vi "createState.vi"(8 "error in (no error)":errorcluster, 10 "State:":T1, 11 "StateFactory in":refnum<class "StateFactory.lvclass">) -> (0 "error out":errorcluster, 2 "State.lvclass":refnum<class "State.lvclass">, 3 "StateFactory out":refnum<class "StateFactory.lvclass">)   [LabVIEW 2015, in "StateFactory.lvclass"]
uses:
  StateFactory.lvclass
  Typedefs/StateSelector.ctl
  State/State.lvclass
  States/OfflineState/OfflineState.lvclass
  States/FaultState/FaultState.lvclass
  States/StandbyState/StandbyState.lvclass
  States/DisabledState/DisabledState.lvclass
  States/EnabledState/EnabledState.lvclass
  States/WaitForUserInputState/WaitForUserInputState.lvclass
  States/PerformOpenLoopScanState/PerformOpenLoopScanState.lvclass
  States/PerformClosedLoopScanState/PerformClosedLoopScanState.lvclass
  Typedefs/FAMTTypedefs.lvlib
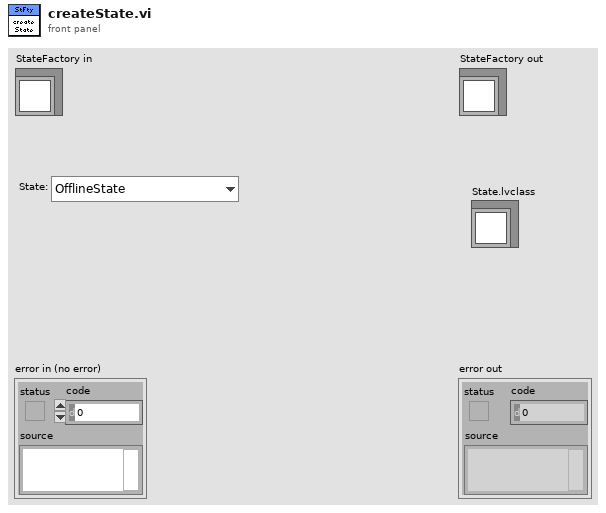
[diagram p1: front panel]
types:
  T1 = typedef "FAMTTypedefs.lvlib/StateSelector.ctl" = enum16{"OfflineState", "FaultState", "StandbyState", "DisabledState", "EnabledState", "WaitForUserInputState", "PerformOpenLoopScanState", "PerformClosedLoopScanState"}
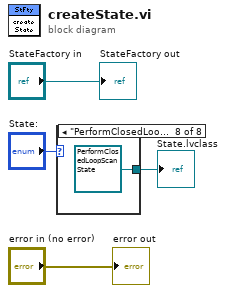
[diagram p0: block diagram]
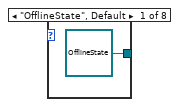
[diagram p2: hidden frame]
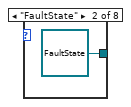
[diagram p3: hidden frame]
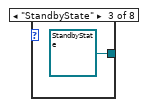
[diagram p4: hidden frame]
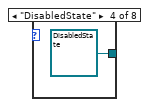
[diagram p5: hidden frame]
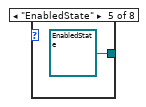
[diagram p6: hidden frame]
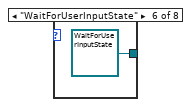
[diagram p7: hidden frame]
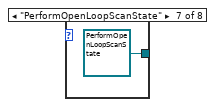
[diagram p8: hidden frame]
diagram:
  n1 = case shown="\"PerformClosedLoopScanState\"" "State:" {
    tunnel: [refnum<class "OfflineState.lvclass"> refnum ("OfflineState.lvclass") refnum<class "FaultState.lvclass"> refnum ("FaultState.lvclass") refnum<class "StandbyState.lvclass"> refnum ("StandbyState.lvclass") refnum<class "DisabledState.lvclass"> refnum ("DisabledState.lvclass") refnum<class "EnabledState.lvclass"> refnum ("EnabledState.lvclass") refnum<class "WaitForUserInputState.lvclass"> refnum ("WaitForUserInputState.lvclass") refnum<class "PerformOpenLoopScanState.lvclass"> refnum ("PerformOpenLoopScanState.lvclass") refnum<class "PerformClosedLoopScanState.lvclass"> refnum ("PerformClosedLoopScanState.lvclass")] -> w1
    frame "OfflineState", Default {
    }
    frame "FaultState" {
    }
    frame "StandbyState" {
    }
    frame "DisabledState" {
    }
    frame "EnabledState" {
    }
    frame "WaitForUserInputState" {
    }
    frame "PerformOpenLoopScanState" {
    }
    frame "PerformClosedLoopScanState" {
    }
  }
  "State.lvclass" <- w1
  "error out" <- "error in (no error)"
  "StateFactory out" <- "StateFactory in"
